vi "RampRate.vi"(8 "error in (no error)":errorcluster, 10 "Ramp rate (A/sec)":dbl format="%#_13g", 11 "PS Driver in":refnum<class "PS Driver.lvclass">) -> (0 "error out":errorcluster, 2 "Ramp rate out (A/s)":dbl format="%#_13g", 3 "PS Driver out":refnum<class "PS Driver.lvclass">)   [LabVIEW 2020, in "PS Driver.lvlib" / "PS Driver.lvclass"]
uses:
  PS Driver.lvclass
  PS Driver.lvclass/PS Driver.ctl
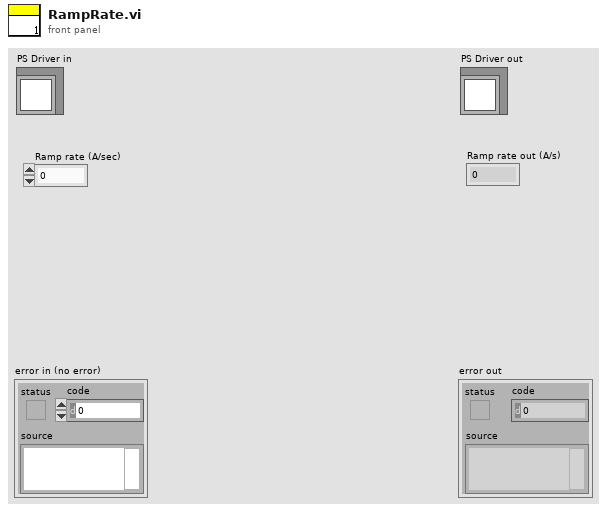
[diagram p1: front panel]
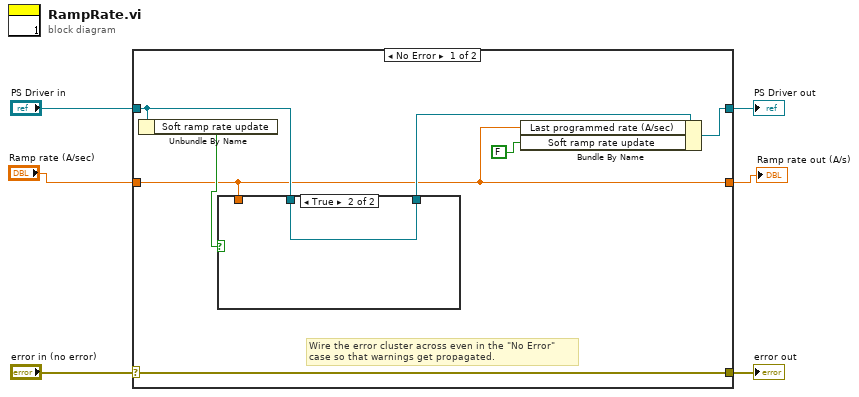
[diagram p0: block diagram]
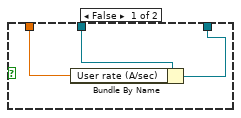
[diagram p2: hidden frame]
diagram:
  n1 = case shown="No Error" "error in (no error)" {
    selector: "error in (no error)" -> [w13 w20]
    tunnel: [w13 w20] -> w5
    tunnel: [w12 w19] -> w3
    tunnel: "PS Driver in" -> [w10 w19]
    tunnel: [w8 w18] -> w2
    tunnel: "Ramp rate (A/sec)" -> [w8 w18]
    frame No Error {
      # "Wire the error cluster across even in the \"No Error\"\ncase so that warnings get propagated."
      n2 = Unbundle By Name(w10) -> ("Soft ramp rate update"=w11:bool)
      n3 = case shown="True" w11 {
        tunnel: w10 -> [w15 w17]
        tunnel: [w14 w17] -> w9
        tunnel: w8 -> [w16 _]
        frame False {
          n4 = Bundle By Name(cluster=w15, "User rate (A/sec)"=w16) -> (w14:refnum<class "PS Driver.lvclass">)
        }
        frame True {
        }
      }
      n5 = Bundle By Name(cluster=w9, "Last programmed rate (A/sec)"=w8, "Soft ramp rate update"=FALSE) -> (w12:refnum<class "PS Driver.lvclass">)
    }
    frame Error {
    }
  }
  "error out" <- w5
  "PS Driver out" <- w3
  "Ramp rate out (A/s)" <- w2
